vi "Grab Hatch Panel in Auto.vi"   [LabVIEW 2018]
uses:
  SubSystems/Hatch Panel Intake/Hatch Panel Intake Global.vi
  SubSystems/Cargo Intake/Cargo Intake Global.vi
  SubSystems/Lift/Lift Global.vi
  SubSystems/Drive Train/Drive Train Global.vi
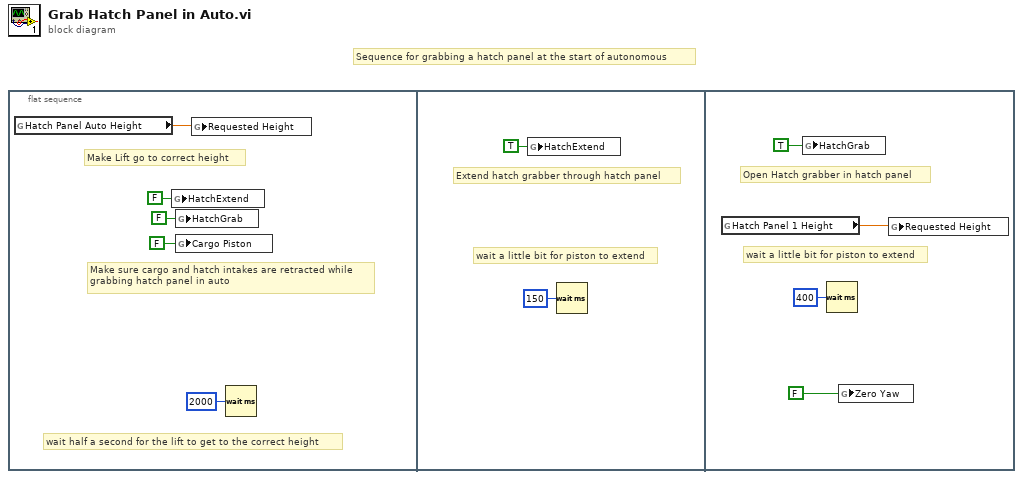
[diagram p0: block diagram]
diagram:
  # "Sequence for grabbing a hatch panel at the start of autonomous"
  n1 = flat-sequence {
    frame #0 {
      # "Make sure cargo and hatch intakes are retracted while\ngrabbing hatch panel in auto"
      # "wait half a second for the lift to get to the correct height"
      # "Make Lift go to correct height"
      n2 = global read "Lift Global.vi" "Hatch Panel Auto Height"() -> (w5:dbl)
      n3 = global write "Hatch Panel Intake Global.vi" "HatchExtend"(FALSE ("HatchExtend")) -> ()
      n4 = global write "Hatch Panel Intake Global.vi" "HatchGrab"(FALSE ("HatchGrab")) -> ()
      n5 = global write "Cargo Intake Global.vi" "Cargo Piston"(FALSE ("Cargo Piston")) -> ()
      n6 = global write "Lift Global.vi" "Requested Height"(w5) -> ()
      n7 = Wait (ms)(milliseconds to wait=u32 2000) -> ()  [unwired: 1 out]
    }
    frame #1 {
      # "wait a little bit for piston to extend"
      # "Extend hatch grabber through hatch panel"
      n8 = global write "Hatch Panel Intake Global.vi" "HatchExtend"(TRUE ("HatchExtend")) -> ()
      n9 = Wait (ms)(milliseconds to wait=u32 150) -> ()  [unwired: 1 out]
    }
    frame #2 {
      # "wait a little bit for piston to extend"
      # "Open Hatch grabber in hatch panel"
      n10 = global read "Lift Global.vi" "Hatch Panel 1 Height"() -> (w8:dbl)
      n11 = global write "Hatch Panel Intake Global.vi" "HatchGrab"(TRUE ("HatchExtend")) -> ()
      n12 = Wait (ms)(milliseconds to wait=u32 400) -> ()  [unwired: 1 out]
      n13 = global write "Drive Train Global.vi" "Zero Yaw"(FALSE ("Reset Field Position")) -> ()
      n14 = global write "Lift Global.vi" "Requested Height"(w8) -> ()
    }
  }
